vi "Steering Motor Controler.vi"   [LabVIEW 2010]
uses:
  Motor Output Global.vi
  Motor Encoder Global.vi
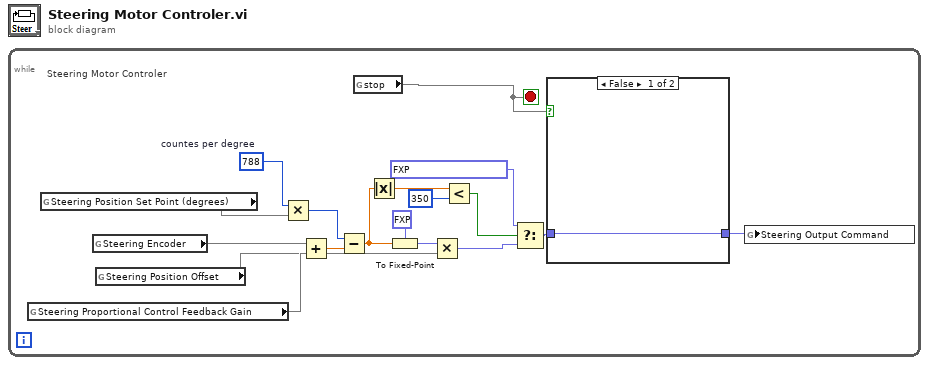
[diagram p0: block diagram]
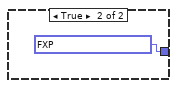
[diagram p2: hidden frame]
diagram:
  n1 = while {
    stop <- w14 stop-if-true
    w12 = 788  # countes per degree
    # "Steering Motor Controler"
    n2 = global read "Motor Encoder Global.vi" "Steering Proportional Control Feedback Gain"() -> (w13)
    n3 = global read "Motor Encoder Global.vi" "Steering Position Set Point (degrees)"() -> (w9)
    n4 = global read "Motor Encoder Global.vi" "Steering Encoder"() -> (w15)
    n5 = global read "Motor Encoder Global.vi" "Steering Position Offset"() -> (w11)
    n6 = Multiply(x=w12, y=w9) -> (x*y=w10:i32)
    n7 = Add(x=w15, y=w11) -> (x+y=w18:dbl)
    n8 = Subtract(x=w10, y=w18) -> (x-y=w7:dbl)
    n9 = global read "Motor Encoder Global.vi" "stop"() -> (w14)
    n10 = Absolute Value(x=w7) -> (abs(x)=w1:dbl)
    n11 = To Fixed-Point(fixed-point type=fxp<+/-,20,5> 0.0, number=w7) -> (fixed-point=w8:fxp<+/-,20,5>)
    n12 = Multiply(x=w8, y=w13) -> (x*y=w5:fxp<+/-,20,5>)
    n13 = Less?(x=w1, y=350) -> (x < y?=w4:bool)
    n14 = Select(t=fxp<+/-,20,5> 0.0, s=w4, f=w5) -> (s? t:f=w2:fxp<+/-,20,5>)
    n15 = case shown="False" w14 {
      tunnel: [w19 fxp<+/-,20,5> 0.0] -> w16
      tunnel: w2 -> [w19 _]
      frame False {
      }
      frame True {
      }
    }
    n16 = global write "Motor Output Global.vi" "Steering Output Command"(w16) -> ()
  }
